vi "QueueObtainer.vi"(8 "error in (no error)":errorcluster) -> (0 "error out":errorcluster, 3 "queue out":refnum<queue>)   [LabVIEW 2014]
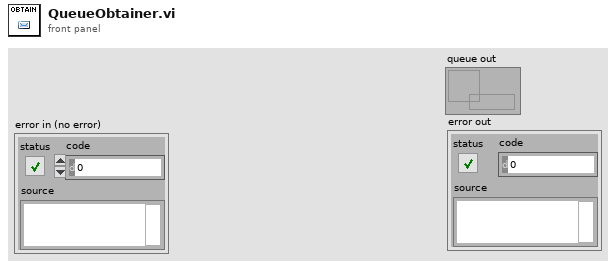
[diagram p1: front panel]
types:
  T1 = cluster{"Message":string, "Message Data":variant}
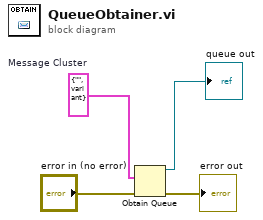
[diagram p0: block diagram]
diagram:
  w4 = T1 {"Message"="", "Message Data"=variant}  # Message Cluster
  n1 = Obtain Queue(element data type=w4, error in (no error)="error in (no error)") -> (queue out=→"queue out":refnum<queue>, error out=→"error out":errorcluster)  [unwired: 3 in, 1 out]
